vi "Remove Header.vi"(8 "error in":errorcluster, 10 "header":string, 11 "net-http-client in":refnum<class "net-http-client.lvclass">) -> (0 "error out":errorcluster, 3 "net-http-client out":refnum<class "net-http-client.lvclass">)   [LabVIEW 2020, in "net-http-client.lvclass"]
uses:
  net-http-client.lvclass
  net-http-client.lvclass/net-http-client.ctl
  <vilib>/Viviota/Viviota HTTP Client NET/HTTPHeaders_NET/HttpHeaders_NET.lvclass
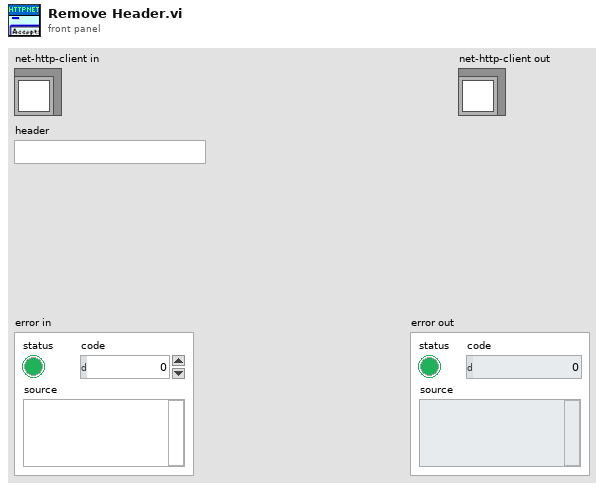
[diagram p1: front panel]
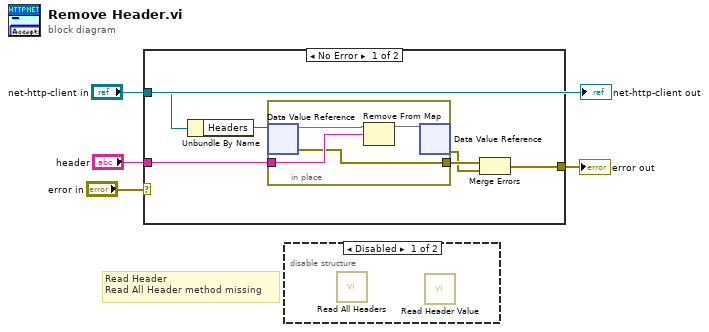
[diagram p0: block diagram]
diagram:
  # "Read Header\nRead All Header method missing"
  n1 = case shown="No Error" "error in" {
    selector: "error in" -> [_ w15]
    tunnel: "net-http-client in" -> [w10 _]
    tunnel: "header" -> [w8 _]
    tunnel: [w5 w15] -> w1
    frame No Error {
      n2 = Unbundle By Name(w10) -> ("Headers"=w9:refnum<data-value>)
      n3 = in-place {
        in-place-border: w8 -> [w13]
        in-place-border: [w11] -> w7
        n4 = in-place-dvr #1(w9) -> (w14:map{string, string}, w11:errorcluster)
        n5 = Remove From Map(10:w13, 11:w14) -> (3:w12:map{string, string})  [unwired: 2 out]
        n6 = in-place-dvr #1(w12) -> (w6:errorcluster)  [unwired: 1 out]
      }
      n7 = Merge Errors(w7, w6) -> (w5:errorcluster)
    }
    frame Error {
    }
  }
  "error out" <- w1
  n8 = disable-structure shown="Disabled" {
    frame Disabled {
      n9 = call-dynamic "Read All Headers.vi"() -> ()  [unwired: 8 in, 4 out]
      n10 = call-dynamic "Read Header Value.vi"() -> ()  [unwired: 7 in, 5 out]
    }
    frame Enabled {
    }
  }
  "net-http-client out" <- "net-http-client in"
